vi "AverageSamples.vi"(1 "data":dbl[][](array[numeric])) -> (0 "Array":dbl[](array[numeric]))   [LabVIEW 2013]
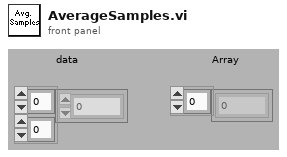
[diagram p1: front panel]
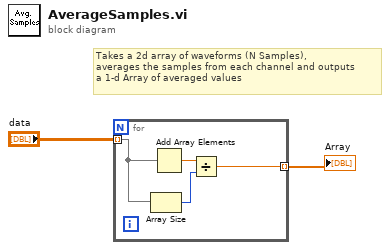
[diagram p0: block diagram]
diagram:
  # "Takes a 2d array of waveforms (N Samples),\naverages the samples from each channel and outputs \na 1-d Array of averaged values"
  n1 = for {
    tunnel: "data" -> [w5] mode=indexing
    tunnel: [w3] -> w2 mode=indexing
    n2 = Array Size(array=w5) -> (size(s)=w4:i32)
    n3 = Add Array Elements(numeric array=w5) -> (sum=w6:dbl)
    n4 = Divide(x=w6, y=w4) -> (x/y=w3:dbl)
  }
  "Array" <- w2
